vi "Probe RawData.vi"(3 "Error In":errorcluster, 4 "Raw Data":i8[](array[numeric]), 5 "DIMActor":refnum<class "DIMActor.lvclass">) -> (0 "Error Out":errorcluster)   [LabVIEW 2012, in "DIMActor.lvlib" / "DIMActor.lvclass"]
doc: "Probe DIM raw data."
uses:
  DIMActor.lvclass
  <vilib>/Utility/miscctls.llb/LVDateTimeRec.ctl
  SVN/LV2009/GPL/lib.lib/DimLVEvent/LVDimInterface/LVDimInterface.lvlib
panel:
  out "date time rec":T1
  out "no link":bool
  out "refNum":u32
  out "serviceID":u32
  out "refNumType":i32
  out "callBackType":i32
  out "typeDescriptor":string
  out "serviceName":string
  out "callBackID (out)":i32
  out "quality":i32
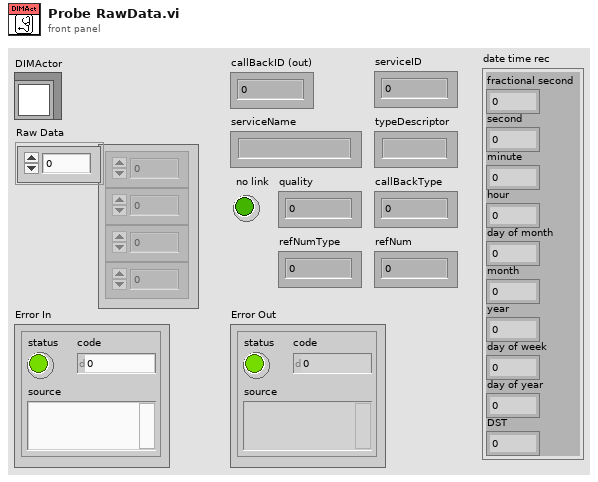
[diagram p1: front panel]
types:
  T1 = typedef "LVDateTimeRec.ctl" = cluster{"fractional second":dbl, "second":i32, "minute":i32, "hour":i32, "day of month":i32, "month":i32, "year":i32, "day of week":i32, "day of year":i32, "DST":i32}
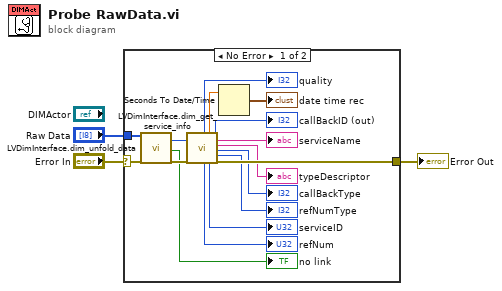
[diagram p0: block diagram]
diagram:
  n1 = case shown="No Error" "Error In" {
    selector: "Error In" -> [w15 w20]
    tunnel: "Raw Data" -> [w19 _]
    tunnel: [w17 w20] -> w2
    frame No Error {
      n2 = call "LVDimInterface.dim_unfold_data.vi"("rawData"=w19, "error in (no error)"=w15) -> ("callBackID"=w16:i32, "no link"=→"no link":bool, "error out"=w18:errorcluster)  [unwired: 14 in, 1 out]
      n3 = call "LVDimInterface.dim_get_service_info.vi"("callBackID"=w16, "error in (no error)"=w18) -> ("quality"=→"quality":i32, "refNum"=→"refNum":u32, "timeStamp"=w14:dbl, "serviceID"=→"serviceID":u32, "callBackID (out)"=→"callBackID (out)":i32, "serviceName"=→"serviceName":string, "typeDescriptor"=→"typeDescriptor":string, "callBackType"=→"callBackType":i32, "refNumType"=→"refNumType":i32, "error out"=w17:errorcluster)  [unwired: 8 in]
      n4 = Seconds To Date/Time(time stamp (now)=w14) -> (date time rec=→"date time rec":T1)  [unwired: 1 in]
    }
    frame Error {
    }
  }
  "Error Out" <- w2
